vi "AcceControl.vi"(8 "dt":dbl, 10 "TempAngle":dbl format="%#_13g", 11 "angle sample":dbl) -> (0 "temp angle out":dbl, 3 "control out":dbl)   [LabVIEW 2014]
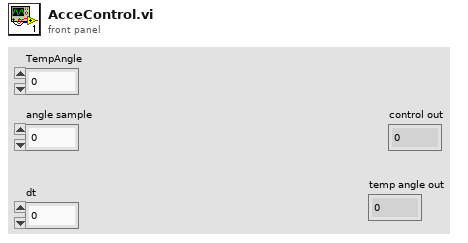
[diagram p1: front panel]
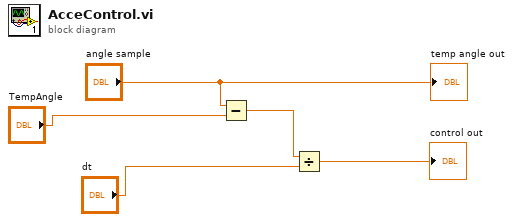
[diagram p0: block diagram]
diagram:
  n1 = Subtract(x="angle sample", y="TempAngle") -> (x-y=w5:dbl)
  n2 = Divide(x=w5, y="dt") -> (x/y=→"control out":dbl)
  "temp angle out" <- "angle sample"
